vi "initialise.vi"(8 "error in (no error)":errorcluster, 11 "GenericTrajectory in":refnum<class "TrajectoryDL110420DoubleCircle.lvclass">) -> (0 "error out":errorcluster, 3 "GenericTrajectory out":refnum<class "TrajectoryDL110420DoubleCircle.lvclass">)   [LabVIEW 2010, in "TrajectoryDL110420DoubleCircle.lvclass"]
uses:
  TrajectoryDL110420DoubleCircle.lvclass
  TrajectoryDL091126GenericVoxel/TrajectoryDL091126GenericVoxel/TrajectoryDL091126GenericVoxel.lvclass
  common/enumerations/x_y_z_enumeration.ctl
  common/enumerations/functional_global_action_enum.ctl
  TrajectoryDL110420DoubleCircle.lvclass/TrajectoryDL110420DoubleCircle.ctl
  common/classes/ImageCollection/ImageCollection/ImageCollection.lvclass
  common/classes/Image/Image/Image.lvclass
  common/classes/SpaceVector/SpaceVector/SpaceVector.lvclass
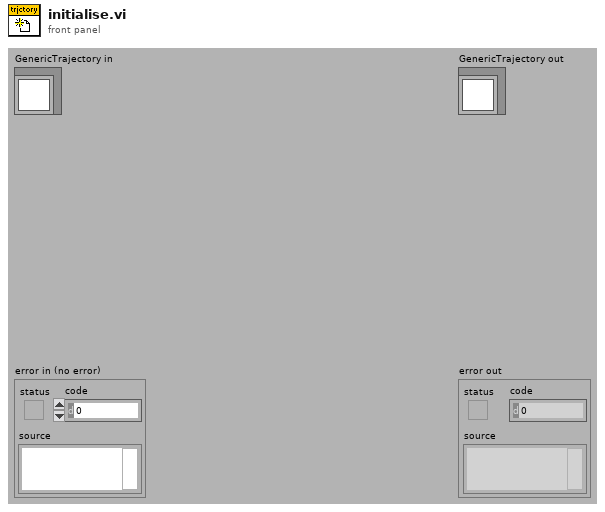
[diagram p1: front panel]
types:
  T1 = typedef "x_y_z_enumeration.ctl" = enum16{"x", "y", "z"}
  T2 = typedef "functional_global_action_enum.ctl" = enum16{"get", "set", "reset"}
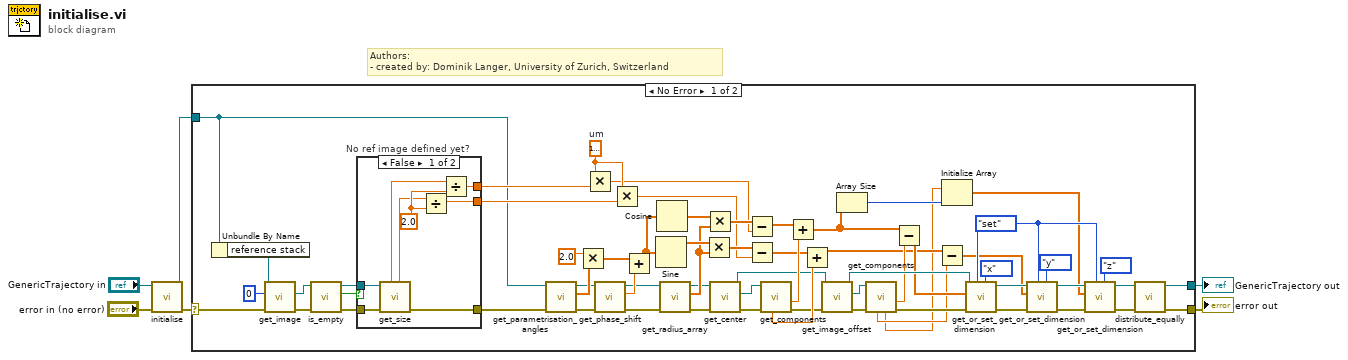
[diagram p0: block diagram]
diagram:
  # "Authors: \n- created by: Dominik Langer, University of Zurich, Switzerland"
  n1 = call-parent "initialise.vi"("error in (no error)"="error in (no error)", "GenericTrajectory in"="GenericTrajectory in") -> ("error out"=w4:errorcluster, "GenericTrajectory out"=w3:refnum<class "TrajectoryDL110420DoubleCircle.lvclass">)  [unwired: 8 in]
  n2 = case shown="No Error" w4 {
    selector: w4 -> [w60 w80]
    tunnel: w3 -> [w11 w81]
    tunnel: [w7 w81] -> w2
    tunnel: [w9 w80] -> w1
    frame No Error {
      w32 = dbl[unit] 1e-06  # um
      w64 = functional_global_action_enum."set" ("action")
      n3 = Unbundle By Name(w11) -> ("reference stack"=w62:refnum<class "ImageCollection.lvclass">)
      n4 = call-dynamic "get_image.vi"("error in (no error)"=w60, "index"=0, "ImageCollection in"=w62) -> ("error out"=w59:errorcluster, "Image.lvclass"=w57:refnum<class "Image.lvclass">)  [unwired: 6 in, 1 out]
      n5 = call-dynamic "is_empty.vi"("error in (no error)"=w59, "Image in"=w57) -> ("error out"=w58:errorcluster, "emtpy?"=w55:bool, "Image out"=w56:refnum<class "Image.lvclass">)  [unwired: 7 in]
      n6 = case "No ref image defined yet?" shown="False" w55 {
        tunnel: [w78 w79] -> w12
        tunnel: [w75 _] -> w34
        tunnel: [w73 _] -> w33
        tunnel: w58 -> [w72 w79]
        tunnel: w56 -> [w71 _]
        frame False {
          w77 = 2.0 ("y")
          n7 = call-dynamic "get_size.vi"("error in (no error)"=w72, "Image in"=w71) -> ("error out"=w78:errorcluster, "physical size y"=w74:dbl, "physical size x"=w76:dbl)  [unwired: 2 in, 5 out]
          n8 = Divide(x=w74, y=w77) -> (x/y=w73:dbl)
          n9 = Divide(x=w76, y=w77) -> (x/y=w75:dbl)
        }
        frame True {
        }
      }
      n10 = call-dynamic "get_parametrisation_angles.vi"("error in (no error)"=w12, "TrajectoryDL110420DoubleCircle in"=w11) -> ("error out"=w49:errorcluster, "angles"=w54:dbl[], "TrajectoryDL110420DoubleCircle out"=w48:refnum<class "TrajectoryDL110420DoubleCircle.lvclass">)  [unwired: 7 in]
      n11 = Multiply(x=2.0, y=w54) -> (x*y=w51:dbl[])
      n12 = Multiply(x=w32, y=w34) -> (x*y=w29:dbl[unit])
      n13 = call-dynamic "get_phase_shift.vi"("error in (no error)"=w49, "TrajectoryDL110420DoubleCircle in"=w48) -> ("error out"=w44:errorcluster, "phase shift"=w52:dbl, "TrajectoryDL110420DoubleCircle out"=w43:refnum<class "TrajectoryDL110420DoubleCircle.lvclass">)  [unwired: 7 in]
      n14 = Multiply(x=w32, y=w33) -> (x*y=w26:dbl[unit])
      n15 = Add(x=w51, y=w52) -> (x+y=w50:dbl[])
      n16 = Sine(x=w50) -> (sin(x)=w47:dbl[])
      n17 = Cosine(x=w50) -> (cos(x)=w46:dbl[])
      n18 = call-dynamic "get_radius_array.vi"("error in (no error)"=w44, "TrajectoryDL110420DoubleCircle in"=w43) -> ("error out"=w42:errorcluster, "radius array"=w45:dbl[unit][], "TrajectoryDL110420DoubleCircle out"=w41:refnum<class "TrajectoryDL110420DoubleCircle.lvclass">)  [unwired: 7 in]
      n19 = Multiply(x=w47, y=w45) -> (x*y=w28:dbl[unit][])
      n20 = Multiply(x=w46, y=w45) -> (x*y=w31:dbl[unit][])
      n21 = call-dynamic "get_center.vi"("error in (no error)"=w42, "TrajectoryDL110420DoubleCircle in"=w41) -> ("error out"=w40:errorcluster, "center"=w39:refnum<class "SpaceVector.lvclass">, "TrajectoryDL110420DoubleCircle out"=w24:refnum<class "TrajectoryDL110420DoubleCircle.lvclass">)  [unwired: 7 in]
      n22 = Subtract(x=w31, y=w29) -> (x-y=w30:dbl[unit][])
      n23 = Subtract(x=w28, y=w26) -> (x-y=w27:dbl[unit][])
      n24 = call "get_components.vi"("error in (no error)"=w40, "SpaceVector in"=w39) -> ("error out"=w25:errorcluster, "x"=w38:dbl[unit], "y"=w37:dbl[unit])  [unwired: 4 in, 3 out]
      n25 = Add(x=w30, y=w38) -> (x+y=w19:dbl[unit][])
      n26 = Add(x=w27, y=w37) -> (x+y=w16:dbl[unit][])
      n27 = call-dynamic "get_image_offset.vi"("error in (no error)"=w25, "TrajectoryDL110420DoubleCircle in"=w24) -> ("error out"=w22:errorcluster, "offset"=w20:refnum<class "SpaceVector.lvclass">, "TrajectoryDL110420DoubleCircle out"=w23:refnum<class "TrajectoryDL110420DoubleCircle.lvclass">)  [unwired: 7 in]
      n28 = Array Size(array=w19) -> (size(s)=w36:i32)
      n29 = call "get_components.vi"("error in (no error)"=w22, "SpaceVector in"=w20) -> ("error out"=w21:errorcluster, "x"=w18:dbl[unit], "z"=w13:dbl[unit], "y"=w14:dbl[unit])  [unwired: 4 in, 2 out]
      n30 = Subtract(x=w19, y=w18) -> (x-y=w17:dbl[unit][])
      n31 = Subtract(x=w16, y=w14) -> (x-y=w15:dbl[unit][])
      n32 = Initialize Array(w13, w36) -> (w35:dbl[unit][])
      n33 = call-dynamic "get_or_set_dimension.vi"("dimension"=x_y_z_enumeration."x", "action"=w64, "error in (no error)"=w21, "pixel values in (single dimension)"=w17, "GenericTrajectory in"=w23) -> ("error out"=w70:errorcluster, "GenericTrajectory out"=w69:refnum<class "TrajectoryDL110420DoubleCircle.lvclass">)  [unwired: 4 in, 1 out]
      n34 = call-dynamic "get_or_set_dimension.vi"("dimension"=x_y_z_enumeration."y", "action"=w64, "error in (no error)"=w70, "pixel values in (single dimension)"=w15, "GenericTrajectory in"=w69) -> ("error out"=w65:errorcluster, "GenericTrajectory out"=w66:refnum<class "TrajectoryDL110420DoubleCircle.lvclass">)  [unwired: 4 in, 1 out]
      n35 = call-dynamic "get_or_set_dimension.vi"("dimension"=x_y_z_enumeration."z", "action"=w64, "error in (no error)"=w65, "pixel values in (single dimension)"=w35, "GenericTrajectory in"=w66) -> ("error out"=w10:errorcluster, "GenericTrajectory out"=w8:refnum<class "TrajectoryDL110420DoubleCircle.lvclass">)  [unwired: 4 in, 1 out]
      n36 = call-dynamic "distribute_equally.vi"("error in (no error)"=w10, "TrajectoryDL091126GenericVoxel in"=w8) -> ("error out"=w9:errorcluster, "TrajectoryDL091126GenericVoxel out"=w7:refnum<class "TrajectoryDL110420DoubleCircle.lvclass">)  [unwired: 7 in, 1 out]
    }
    frame Error {
    }
  }
  "error out" <- w1
  "GenericTrajectory out" <- w2
